vi "MeasureRMS.vi"(6 "error in":errorcluster, 7 "stop":bool, 9 "input cluster":T1) -> (0 "error out":errorcluster, 1 "data":dynamicdata(graph), 2 "AC estimate (Vrms)":dbl format="%0.2f")   [LabVIEW 2014]
uses:
  <vilib>/Analysis/NI_AALPro.lvlib
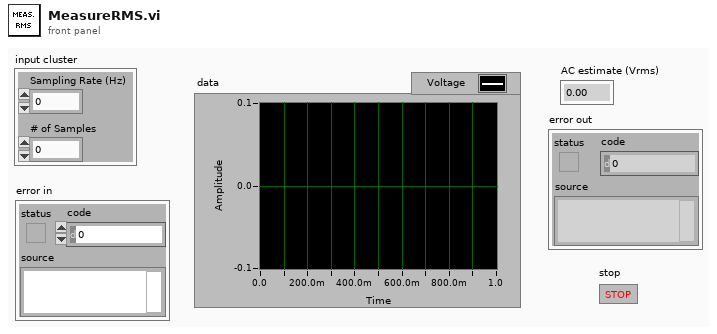
[diagram p1: front panel]
types:
  T1 = cluster{"Sampling Rate (Hz)":dbl, "# of Samples":dbl}
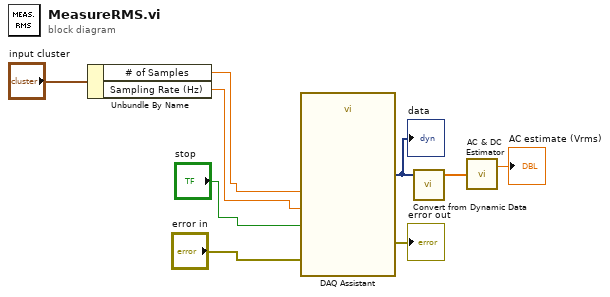
[diagram p0: block diagram]
diagram:
  n1 = Unbundle By Name("input cluster") -> ("# of Samples"=w1:dbl, "Sampling Rate (Hz)"=w2:dbl)
  n2 = call "DAQ Assistant"("rate"=w2, "number of samples"=w1, "error in"="error in", "stop (T)"="stop") -> ("data"=w8:dynamicdata, "error out"=→"error out":errorcluster)  [unwired: 13 in, 1 out]
  "data" <- w8
  n3 = call "Convert from Dynamic Data"("Dynamic Data Type"=w8) -> ("Array"=w5:dbl[])  [unwired: 3 in]
  n4 = call <vilib>:"AC & DC Estimator.vi"("Signal (V)"=w5) -> ("AC estimate (Vrms)"=→"AC estimate (Vrms)":dbl)  [unwired: 1 out]
